vi "LabVIEW Vending Machine.vi"() -> ()   [LabVIEW 2017]
uses:
  VendingMachineStates.ctl
panel:
  in  "Dime":bool
  in  "Nickel":bool
  in  "Quarter":bool
  in  "stop":bool
  out "Message to User":string
  out "Change Returned":dbl format="%.2f"
  in  "Pepsi":bool
  in  "Coke":bool
  out "Coke Display":u16(ring)
  in  "Return Change":bool
  out "Value Deposited":dbl format="%.2f"
  # "$0.75"
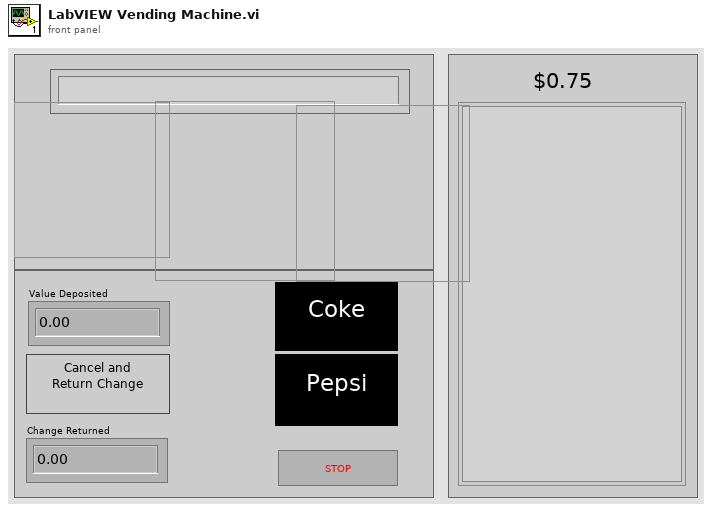
[diagram p1: front panel]
types:
  T1 = typedef "VendingMachineStates.ctl" = enum16{"Initialize", "Insert Coin", "Coke Disp", "Pepsi Disp", "Cancel", "Stop"}
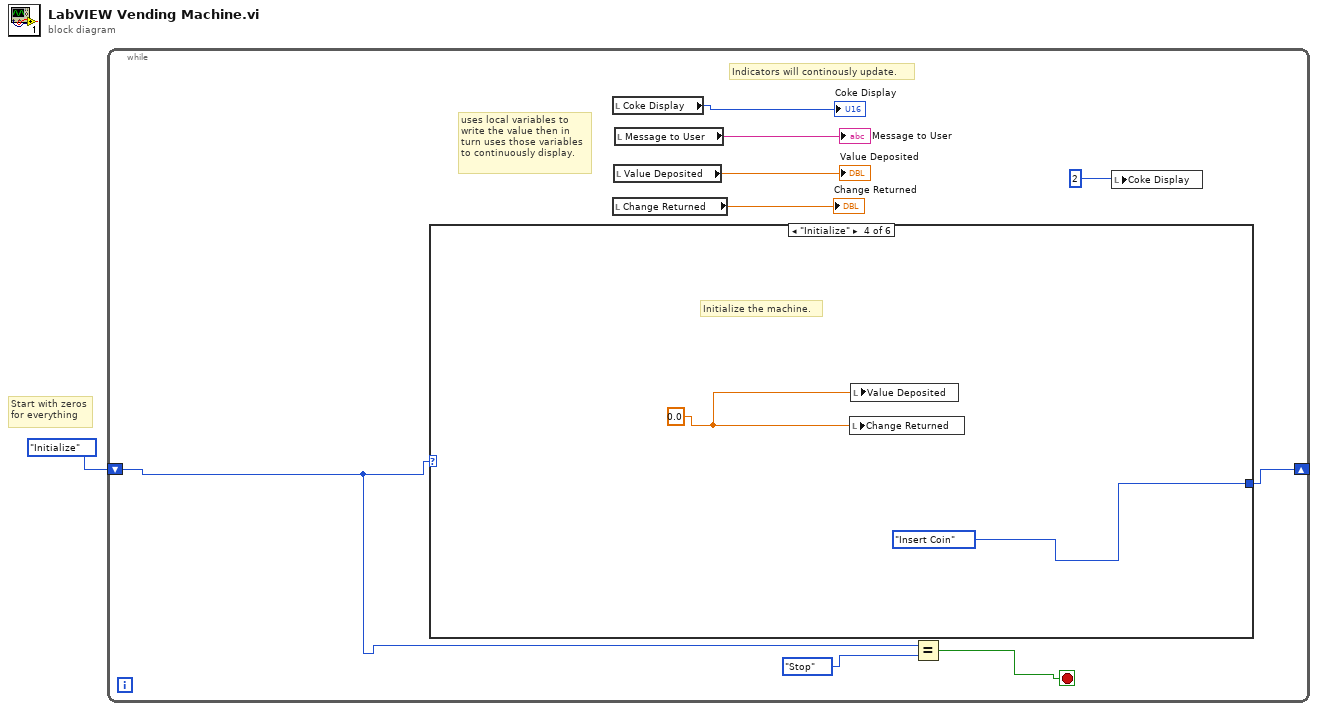
[diagram p0: block diagram]
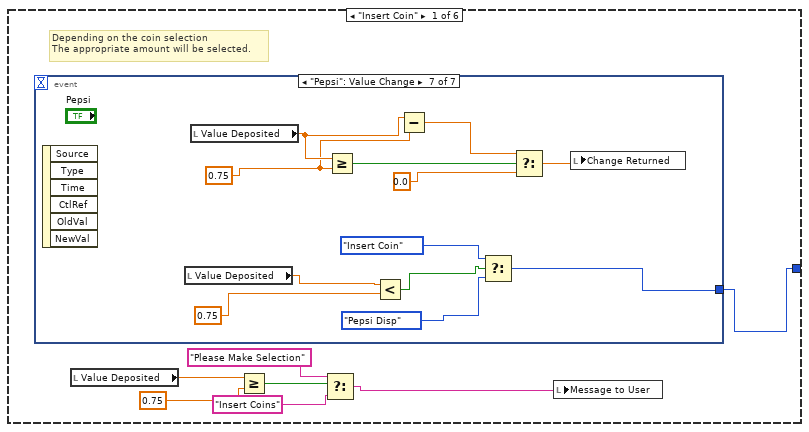
[diagram p2: hidden frame]
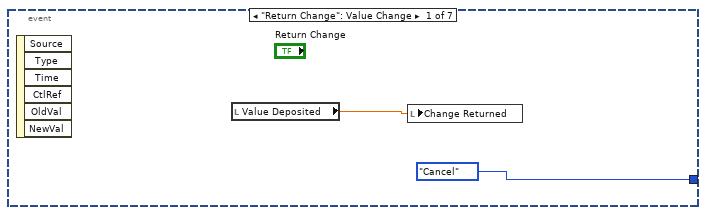
[diagram p3: hidden frame]
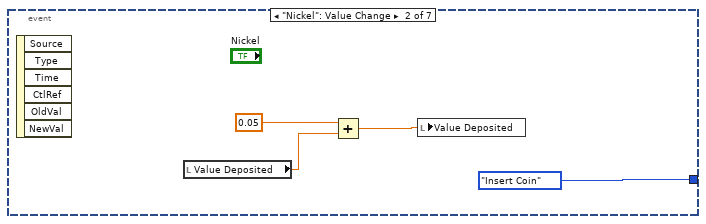
[diagram p4: hidden frame]
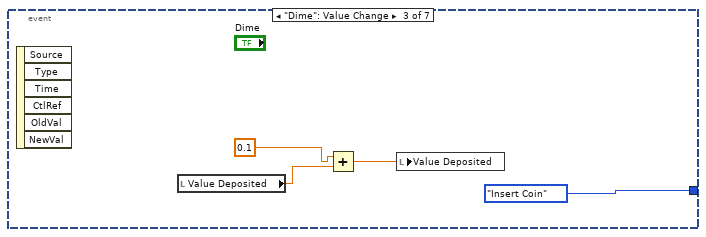
[diagram p5: hidden frame]
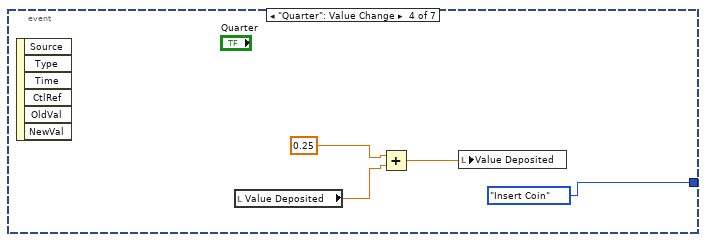
[diagram p6: hidden frame]
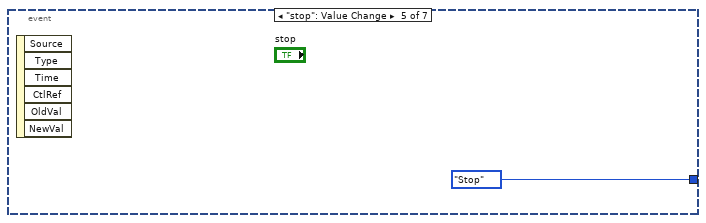
[diagram p7: hidden frame]
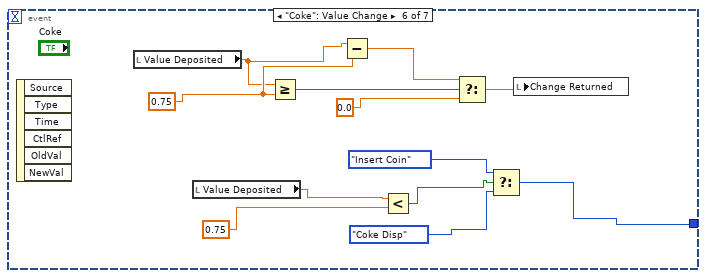
[diagram p8: hidden frame]
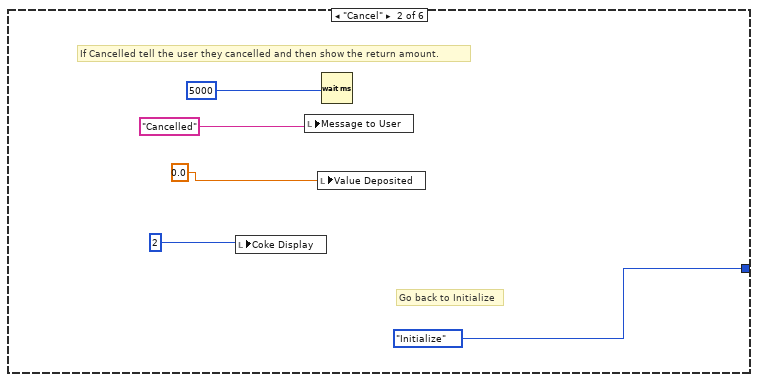
[diagram p9: hidden frame]
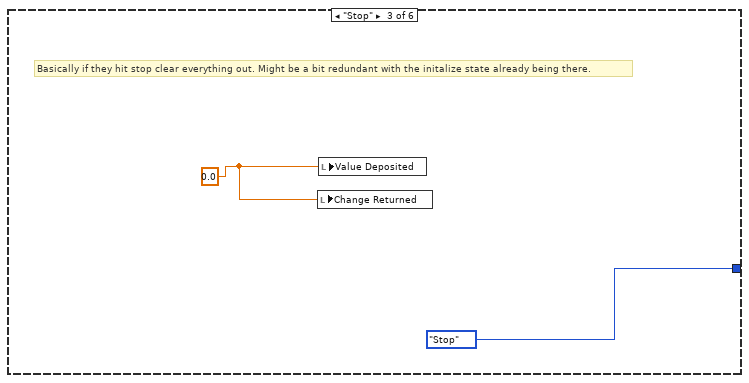
[diagram p10: hidden frame]
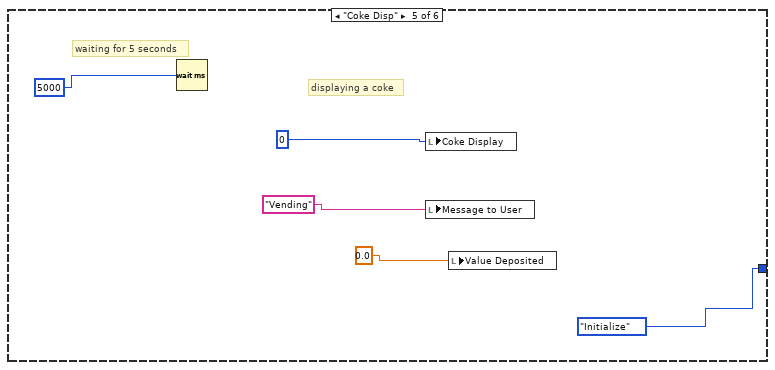
[diagram p11: hidden frame]
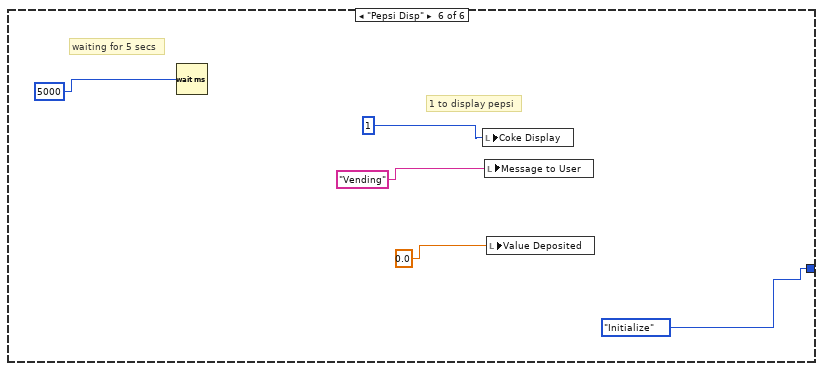
[diagram p12: hidden frame]
diagram:
  # "Start with zeros\nfor everything"
  n1 = while {
    shift-right: [w3] -> _
    shift-left: VendingMachineStates."Initialize" -> [w2]
    stop <- w9 stop-if-true
    # "uses local variables to \nwrite the value then in \nturn uses those variables\nto continuously display."
    # "Indicators will continously update."
    n2 = case shown="\"Initialize\"" w2 {
      tunnel: [w17 VendingMachineStates."Initialize" VendingMachineStates."Stop" VendingMachineStates."Insert Coin" VendingMachineStates."Initialize" VendingMachineStates."Initialize"] -> w3
      frame "Insert Coin" {
        # "Depending on the coin selection\nThe appropriate amount will be selected."
        n3 = event shown="[6] \"Pepsi\": Value Change" {
          selector: _ -> [_ _ _ _ _ _ _]
          dyn-events: _ -> [_ _ _ _ _ _ _]
          timeout: _ -> [_ _ _ _ _ _ _]
          tunnel: [VendingMachineStates."Cancel" VendingMachineStates."Insert Coin" VendingMachineStates."Insert Coin" VendingMachineStates."Insert Coin" VendingMachineStates."Stop" w39 w56] -> w17
          event "Return Change": Value Change {
            n4 = event-data() -> ()  [unwired: 1 in, 6 out]
            n5 = local read "Value Deposited"() -> (w18:dbl)
            n6 = local write "Change Returned"(w18) -> ()
          }
          event "Nickel": Value Change {
            n7 = event-data() -> ()  [unwired: 1 in, 6 out]
            n8 = local read "Value Deposited"() -> (w21:dbl)
            n9 = Add(x=0.05, y=w21) -> (x+y=w20:dbl)
            n10 = local write "Value Deposited"(w20) -> ()
          }
          event "Dime": Value Change {
            n11 = event-data() -> ()  [unwired: 1 in, 6 out]
            n12 = local read "Value Deposited"() -> (w26:dbl)
            n13 = Add(x=0.1, y=w26) -> (x+y=w25:dbl)
            n14 = local write "Value Deposited"(w25) -> ()
          }
          event "Quarter": Value Change {
            n15 = event-data() -> ()  [unwired: 1 in, 6 out]
            n16 = local read "Value Deposited"() -> (w30:dbl)
            n17 = Add(x=0.25, y=w30) -> (x+y=w29:dbl)
            n18 = local write "Value Deposited"(w29) -> ()
          }
          event "stop": Value Change {
            n19 = event-data() -> ()  [unwired: 1 in, 6 out]
          }
          event "Coke": Value Change {
            w37 = 0.75
            n20 = event-data() -> ()  [unwired: 1 in, 6 out]
            n21 = local read "Value Deposited"() -> (w33:dbl)
            n22 = local read "Value Deposited"() -> (w44:dbl)
            n23 = Greater Or Equal?(x=w33, y=w37) -> (x >= y?=w38:bool)
            n24 = Subtract(x=w33, y=w37) -> (x-y=w36:dbl)
            n25 = Less?(x=w44, y=0.75) -> (x < y?=w41:bool)
            n26 = Select(t=w36, s=w38, f=0.0) -> (s? t:f=w34:dbl)
            n27 = Select(t=VendingMachineStates."Insert Coin", s=w41, f=VendingMachineStates."Coke Disp") -> (s? t:f=w39:T1)
            n28 = local write "Change Returned"(w34) -> ()
          }
          event "Pepsi": Value Change {
            w48 = 0.75
            n29 = event-data() -> ()  [unwired: 1 in, 6 out]
            n30 = local read "Value Deposited"() -> (w55:dbl)
            n31 = local read "Value Deposited"() -> (w49:dbl)
            n32 = Greater Or Equal?(x=w49, y=w48) -> (x >= y?=w50:bool)
            n33 = Less?(x=w55, y=0.75) -> (x < y?=w52:bool)
            n34 = Subtract(x=w49, y=w48) -> (x-y=w47:dbl)
            n35 = Select(t=VendingMachineStates."Insert Coin", s=w52, f=VendingMachineStates."Pepsi Disp") -> (s? t:f=w56:T1)
            n36 = Select(t=w47, s=w50, f=0.0) -> (s? t:f=w45:dbl)
            n37 = local write "Change Returned"(w45) -> ()
          }
        }
        n38 = local read "Value Deposited"() -> (w16:dbl)
        n39 = Greater Or Equal?(x=w16, y=0.75) -> (x >= y?=w15:bool)
        n40 = Select(t="Please Make Selection", s=w15, f="Insert Coins") -> (s? t:f=w12:string)
        n41 = local write "Message to User"(w12) -> ()
      }
      frame "Cancel" {
        # "Go back to Initialize"
        # "If Cancelled tell the user they cancelled and then show the return amount."
        n42 = local write "Coke Display"(2) -> ()
        n43 = local write "Message to User"("Cancelled") -> ()
        n44 = local write "Value Deposited"(0.0) -> ()
        n45 = Wait (ms)(milliseconds to wait=5000) -> ()  [unwired: 1 out]
      }
      frame "Stop" {
        w62 = 0.0
        # "Basically if they hit stop clear everything out. Might be a bit redundant with the initalize state already being there."
        n46 = local write "Change Returned"(w62) -> ()
        n47 = local write "Value Deposited"(w62) -> ()
      }
      frame "Initialize" {
        w65 = 0.0
        # "Initialize the machine."
        n48 = local write "Change Returned"(w65) -> ()
        n49 = local write "Value Deposited"(w65) -> ()
      }
      frame "Coke Disp" {
        # "waiting for 5 seconds"
        # "displaying a coke"
        n50 = Wait (ms)(milliseconds to wait=5000) -> ()  [unwired: 1 out]
        n51 = local write "Coke Display"(0) -> ()
        n52 = local write "Message to User"("Vending") -> ()
        n53 = local write "Value Deposited"(0.0) -> ()
      }
      frame "Pepsi Disp" {
        # "waiting for 5 secs"
        # "1 to display pepsi"
        n54 = Wait (ms)(milliseconds to wait=5000) -> ()  [unwired: 1 out]
        n55 = local write "Coke Display"(1) -> ()
        n56 = local write "Message to User"("Vending") -> ()
        n57 = local write "Value Deposited"(0.0) -> ()
      }
    }
    n58 = local read "Coke Display"() -> (→"Coke Display":u16)
    n59 = local read "Change Returned"() -> (→"Change Returned":dbl)
    n60 = local read "Value Deposited"() -> (→"Value Deposited":dbl)
    n61 = local read "Message to User"() -> (→"Message to User":string)
    n62 = Equal?(x=w2, y=VendingMachineStates."Stop") -> (x = y?=w9:bool)
    n63 = local write "Coke Display"(2) -> ()
  }
